vi "Controller Error Status FOFB.vi"() -> ()   [LabVIEW 2011, in "Controller Global Variables.lvlib"]
uses:
  Controller Global Variables.lvlib
panel:
  in  "Controller Error Status FOFB":u16
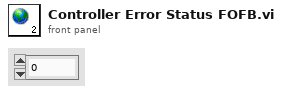
[diagram p1: front panel]
diagram:
